vi "Hatch Grab.vi"(8 "Time":u32, 11 "On/Off":bool) -> ()   [LabVIEW 2018]
uses:
  <vilib>/ErrorRing/Error Ring.xnode
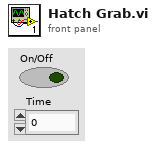
[diagram p1: front panel]
types:
  T1 = typedef "WPI_MotorControlDeviceRef.ctl" = cluster{"DeviceStatus":errorcluster, "Type":T2, "PWM":cluster{"PWM Channel":T3, "DeadBand":T4}, "CAN":cluster{"Device Number":u8, "SetOutput VI Ref":variant, "GetOutput VI Ref":variant, "Enable VI Ref":variant, "Disable VI Ref":variant, "Data":variant}, "Invert":bool, "DIO PWM":cluster{"PWM \"Enable\" Channel":T3, "DIOChannel":T5, "PWM Rate":dbl}}
  T2 = typedef "WPI_MotorControlType.ctl" = enum16{"PWM", "CAN", "DIO PWM"}
  T3 = typedef "FPGA_DIOPWMChannel.ctl" = enum8{"PWM 0", "PWM 1", "PWM 2", "PWM 3", "PWM 4", "PWM 5", "PWM 6", "PWM 7", "PWM 8", "PWM 9", "PWM MXP 0", "PWM MXP 1", "PWM MXP 2", "PWM MXP 3", "PWM MXP 4", "PWM MXP 5", "PWM MXP 6", "PWM MXP 7", "PWM MXP 8", "PWM MXP 9", "Invalid"}
  T4 = typedef "WPI_PWMDeadband.ctl" = cluster{"Name":string, "maxPositivePwm":i32, "minPositivePwm":i32, "centerPwm":i32, "maxNegativePwm":i32, "minNegativePwm":i32, "angularRange":u16}
  T5 = typedef "FPGA_DIOChannel.ctl" = enum8{"DIO 0", "DIO 1", "DIO 2", "DIO 3", "DIO 4", "DIO 5", "DIO 6", "DIO 7", "DIO 8", "DIO 9", "DIO MXP 0", "DIO MXP 1", "DIO MXP 2", "DIO MXP 3", "DIO MXP 4", "DIO MXP 5", "DIO MXP 6", "DIO MXP 7", "DIO MXP 8", "DIO MXP 9", "DIO MXP 10", "DIO MXP 11", "DIO MXP 12", "DIO MXP 13", "DIO MXP 14", "DIO MXP 15", "SPI Port CS1", "SPI Port CS2", "SPI Port CS3", "SPI Port MISO", "SPI Port MOSI", "Invalid"}
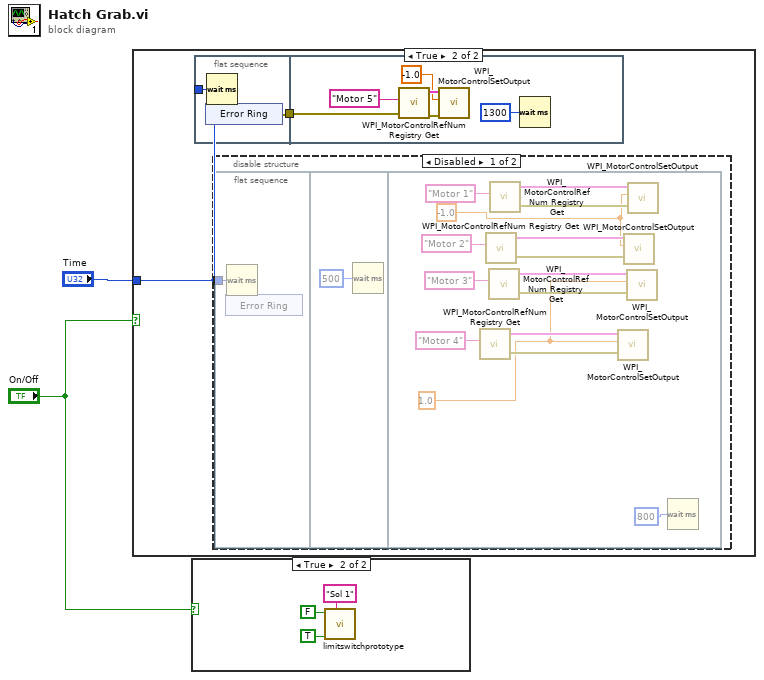
[diagram p0: block diagram]
diagram:
  n1 = case shown="True" "On/Off" {
    tunnel: "Time" -> [_ w3]
    frame False {
    }
    frame True {
      n2 = flat-sequence {
        tunnel: w3 -> [w25]
        tunnel: [w24] -> w4
        tunnel: w4 -> [w29]
        frame #0 {
          n3 = xnode "Error Ring"() -> ("error out"=w24:errorcluster)
          n4 = Wait (ms)(milliseconds to wait=w25) -> ()  [unwired: 1 out]
        }
        frame #1 {
          n5 = call <vilib>:"WPI_MotorControlRefNum Registry Get.vi"("error in (no error)"=w29, "refnum name"="Motor 5") -> ("error out"=w32:errorcluster, "MotorControlDevRef"=w31:T1)  [unwired: 8 in]
          n6 = call <vilib>:"WPI_MotorControlSetOutput.vi"("error in (no error)"=w32, "Output"=-1.0, "MotorControlDevRef"=w31) -> ()  [unwired: 6 in, 3 out]
          n7 = Wait (ms)(milliseconds to wait=u32 1300) -> ()  [unwired: 1 out]
        }
      }
      n8 = disable-structure shown="Disabled" {
        disable-tunnel: w3 -> [w5 _]
        frame Disabled {
          n9 = flat-sequence {
            tunnel: w5 -> [w6]
            frame #0 {
              n10 = xnode "Error Ring"() -> ()  [unwired: 1 out]
              n11 = Wait (ms)(milliseconds to wait=w6) -> ()  [unwired: 1 out]
            }
            frame #1 {
              n12 = Wait (ms)(milliseconds to wait=u32 500) -> ()  [unwired: 1 out]
            }
            frame #2 {
              w9 = -1.0
              w11 = 1.0
              n13 = call <vilib>:"WPI_MotorControlRefNum Registry Get.vi"("refnum name"="Motor 4") -> ("error out"=w14:errorcluster, "MotorControlDevRef"=w13:T1)  [unwired: 9 in]
              n14 = call <vilib>:"WPI_MotorControlRefNum Registry Get.vi"("refnum name"="Motor 2") -> ("error out"=w20:errorcluster, "MotorControlDevRef"=w19:T1)  [unwired: 9 in]
              n15 = call <vilib>:"WPI_MotorControlRefNum Registry Get.vi"("refnum name"="Motor 3") -> ("error out"=w17:errorcluster, "MotorControlDevRef"=w16:T1)  [unwired: 9 in]
              n16 = call <vilib>:"WPI_MotorControlRefNum Registry Get.vi"("refnum name"="Motor 1") -> ("error out"=w23:errorcluster, "MotorControlDevRef"=w22:T1)  [unwired: 9 in]
              n17 = call <vilib>:"WPI_MotorControlSetOutput.vi"("error in (no error)"=w14, "Output"=w11, "MotorControlDevRef"=w13) -> ()  [unwired: 6 in, 3 out]
              n18 = call <vilib>:"WPI_MotorControlSetOutput.vi"("error in (no error)"=w20, "Output"=w9, "MotorControlDevRef"=w19) -> ()  [unwired: 6 in, 3 out]
              n19 = call <vilib>:"WPI_MotorControlSetOutput.vi"("error in (no error)"=w17, "Output"=w11, "MotorControlDevRef"=w16) -> ()  [unwired: 6 in, 3 out]
              n20 = call <vilib>:"WPI_MotorControlSetOutput.vi"("error in (no error)"=w23, "Output"=w9, "MotorControlDevRef"=w22) -> ()  [unwired: 6 in, 3 out]
              n21 = Wait (ms)(milliseconds to wait=u32 800) -> ()  [unwired: 1 out]
            }
          }
        }
        frame Enabled {
        }
      }
    }
  }
  n22 = case shown="True" "On/Off" {
    frame False {
    }
    frame True {
      n23 = call "limitswitchprototype.vi"("Sol Name"="Sol 1", "Close"=TRUE, "Open"=FALSE) -> ()  [unwired: 9 in]
    }
  }
